vi "ex_TreeUpdateValues.vi"(4 "error in (no error)":errorcluster, 7 "Data Object in":refnum<k20>) -> (0 "error out":errorcluster, 1 "Dynamic Data":dynamicdata(waveform), 2 "Values as String array":string[][](array[string]), 3 "Header strings":string[](array[string]))   [LabVIEW 2017]
uses:
  <vilib>/Platform/storage/Storage.llb/Get Property (Storage Refnums).vi
  <vilib>/Platform/storage/Storage.llb/Get Property (Enum).vi
  <vilib>/Platform/storage/lvStorage.llb/_loadWaveform.vi
  <vilib>/Platform/storage/lvStorage.llb/xStorage/xStorageSupp/ErrorOut.vi
  <vilib>/Waveform/WDTOps.llb/WDT Waveform to XY Pairs DBL.vi
  <vilib>/Platform/storage/Storage.llb/Get Property (String).vi
  <vilib>/Platform/storage/Storage.llb/__loadStringChannel.vi
  <vilib>/Platform/storage/Storage.llb/__loadDateTimeChannel.vi
  <vilib>/Platform/storage/lvStorage.llb/xStorage/Get Properties/Get Properties.xnode
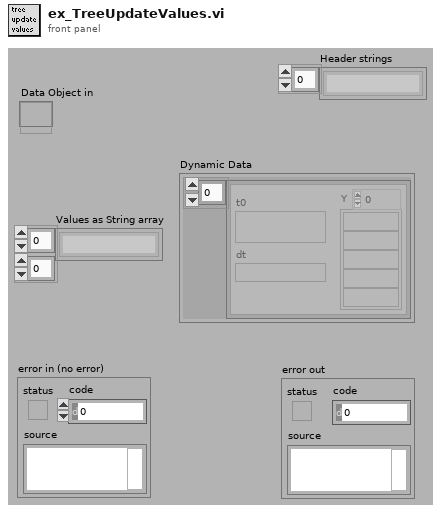
[diagram p1: front panel]
types:
  T1 = enum16{"UPDATE", "READ", "QUERY", "CREATE CHILD", "CREATE", "CONNECT", "DISCONNECT"}
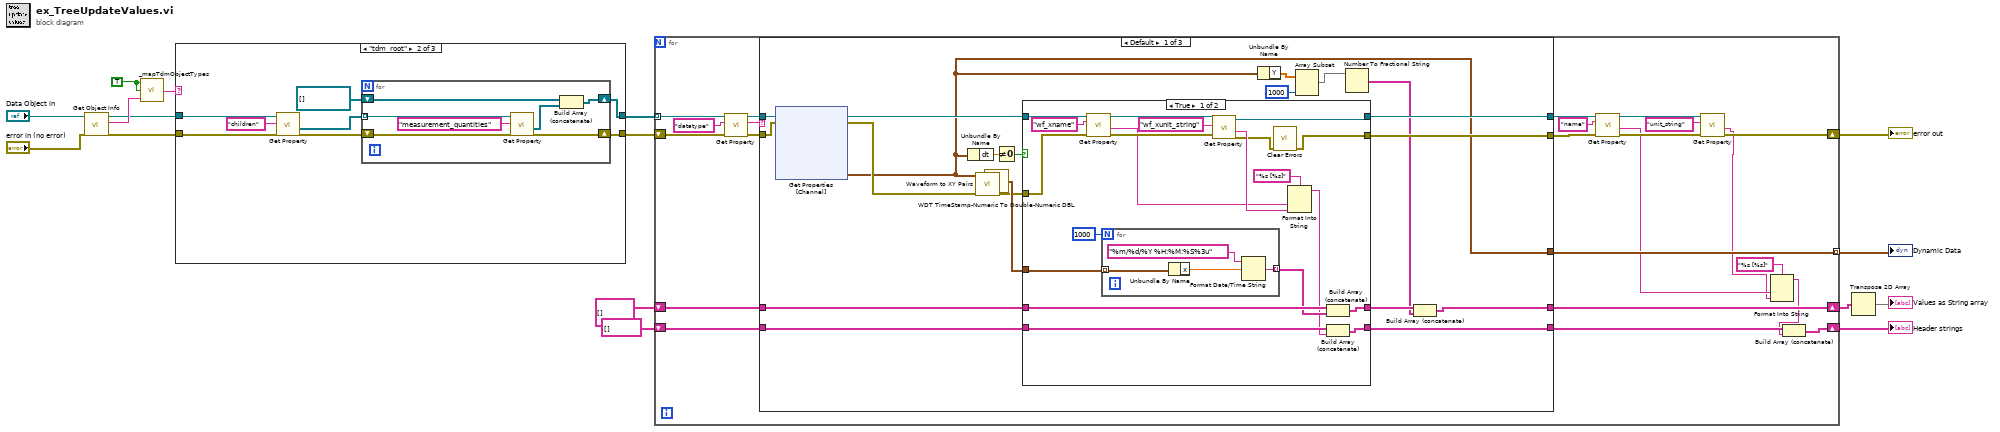
[diagram p0: block diagram]
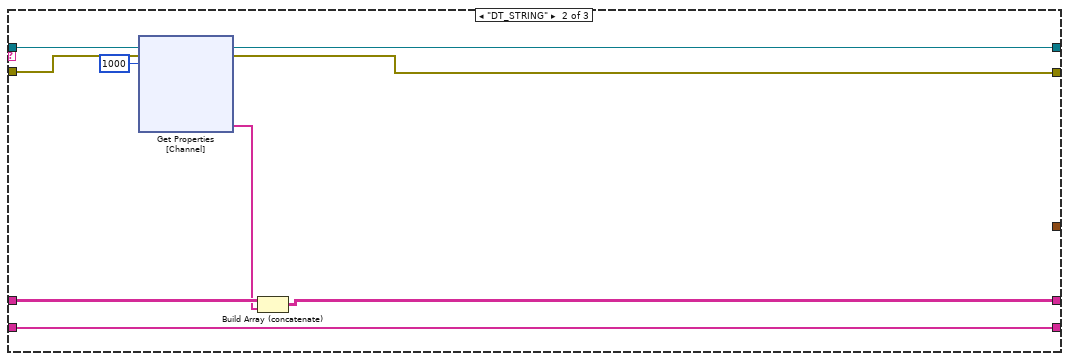
[diagram p3: hidden frame]
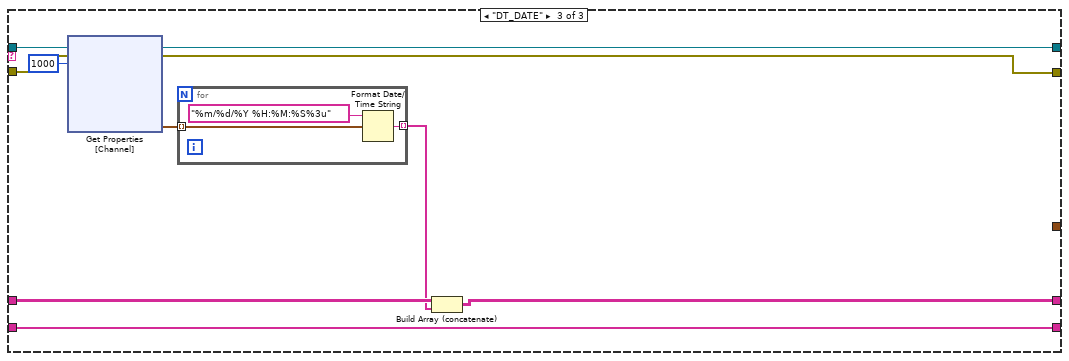
[diagram p4: hidden frame]
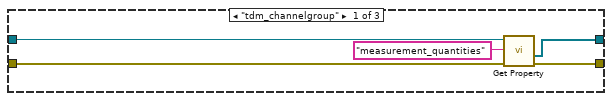
[diagram p5: hidden frame]
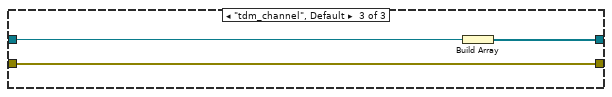
[diagram p6: hidden frame]
diagram:
  w12 = TRUE ("DNL_UnMap?(F)")
  n1 = call <vilib>:"Get Object Info.vi"("error in (no error)"="error in (no error)", "storage refnum"="Data Object in") -> ("error out"=w10:errorcluster, "object type"=w13:string, "storage refnum out"=w8:refnum<k20>)  [unwired: 7 out]
  n2 = call <vilib>:"_mapTdmObjectTypes.vi"(1:w13, "isTdmDataStructure?"=w12, "DNL_UnMap?(F)"=w12) -> (0:w11:string)
  n3 = case shown="\"tdm_root\"" w11 {
    tunnel: w10 -> [w21 w27 w39]
    tunnel: [w19 w29 w39] -> w9
    tunnel: w8 -> [w20 w26 w38]
    tunnel: [w18 w22 w37] -> w6
    frame "tdm_channelgroup" {
      n4 = call-poly <vilib>:"Get Property.vi"("error in (no error)"=w21, "Property name"="measurement_quantities", "storage refnum"=w20) -> ("error out"=w19:errorcluster, "Value"=w18:refnum<k20>[])  [unwired: 7 out]
    }
    frame "tdm_root" {
      n5 = call-poly <vilib>:"Get Property.vi"("error in (no error)"=w27, "Property name"="children", "storage refnum"=w26) -> ("error out"=w25:errorcluster, "Value"=w24:refnum<k20>[])  [unwired: 7 out]
      n6 = for {
        tunnel: w24 -> [w33] mode=indexing
        shift-right: [w30] -> w22
        shift-left: refnum<k20>[] [] ("Value") -> [w32]
        shift-right: [w36] -> w29
        shift-left: w25 -> [w34]
        n7 = call-poly <vilib>:"Get Property.vi"("error in (no error)"=w34, "Property name"="measurement_quantities", "storage refnum"=w33) -> ("error out"=w36:errorcluster, "Value"=w31:refnum<k20>[])  [unwired: 7 out]
        n8 = Build Array (concatenate)(w32, w31) -> (w30:refnum<k20>[])
      }
    }
    frame "tdm_channel", Default {
      n9 = Build Array(w38) -> (w37:refnum<k20>[])
    }
  }
  n10 = for {
    tunnel: [w62] -> w16 mode=indexing
    shift-right: [w44] -> w7
    shift-left: w9 -> [w61]
    tunnel: w6 -> [w56] mode=indexing
    shift-right: [w51] -> w4
    shift-left: string[][] [] -> [w52]
    shift-right: [w48] -> w1
    shift-left: string[] [] -> [w50]
    n11 = call-poly <vilib>:"Get Property.vi"("error in (no error)"=w61, "Property name"="datatype" ("PropertyName"), "storage refnum"=w56) -> ("error out"=w60:errorcluster, "String"=w57:string, "storage refnum out"=w59:refnum<k20>)  [unwired: 6 out]
    n12 = case shown="Default" w57 {
      tunnel: w60 -> [w76 w129 w148]
      tunnel: w59 -> [w77 w128 w147]
      tunnel: [w73 _ _] -> w62
      tunnel: [w79 w127 w146] -> w53
      tunnel: [w78 w126 w145] -> w54
      tunnel: w52 -> [w72 w125 w143]
      tunnel: [w69 w123 w141] -> w51
      tunnel: w50 -> [w65 w121 w139]
      tunnel: [w64 w121 w139] -> w49
      frame Default {
        n13 = xnode "Get Properties\n[Channel]"("storage refnum"=w77, "error in"=w76) -> ("Signal"=w73:waveform(dbl), "storage refnum out"=w75:refnum<k20>, "error out"=w74:errorcluster)  [unwired: 2 out]
        n14 = Unbundle By Name(w73) -> ("dt"=w82:dbl)
        n15 = call-poly <vilib>:"Waveform to XY Pairs.vi"("error in (no error)"=w74, "waveform in"=w73) -> ("error out"=w80:errorcluster, "XY pairs"=w63:cluster{"x":timestamp, "y":dbl}[])  [unwired: 8 out]
        n16 = call <vilib>:"WDT TimeStamp-Numeric To Double-Numeric DBL.vi"("XY pairs w/timestamp time"=w63) -> ("XY pairs w/double time"=w83:cluster{"x":dbl, "y":dbl}[])
        n17 = Not Equal To 0?(x=w82) -> (x != 0?=w81:bool)
        n18 = case shown="True" w81 {
          tunnel: w83 -> [w112 _]
          tunnel: w75 -> [w102 w120]
          tunnel: w80 -> [w101 w119]
          tunnel: [w97 w120] -> w79
          tunnel: [w93 w119] -> w78
          tunnel: w72 -> [w110 w118]
          tunnel: [w111 w118] -> w71
          tunnel: w65 -> [w107 w117]
          tunnel: [w106 w117] -> w64
          frame True {
            n19 = call-poly <vilib>:"Get Property.vi"("error in (no error)"=w101, "Property name"="wf_xname" ("PropertyName"), "storage refnum"=w102) -> ("error out"=w100:errorcluster, "Value"=w95:string, "storage refnum out"=w99:refnum<k20>)  [unwired: 6 out]
            n20 = for {
              N: 1000 -> [_]
              tunnel: w112 -> [w116] mode=indexing
              tunnel: [w113] -> w109 mode=indexing
              n21 = Unbundle By Name(w116) -> ("x"=w114:dbl)
              n22 = Format Date/Time String(time format string (%c)="%m/%d/%Y %H:%M:%S%3u", seconds (now)=w114) -> (date/time string=w113:string)  [unwired: 1 out]
            }
            n23 = call-poly <vilib>:"Get Property.vi"("error in (no error)"=w100, "Property name"="wf_xunit_string" ("PropertyName"), "storage refnum"=w99) -> ("error out"=w94:errorcluster, "Value"=w96:string, "storage refnum out"=w97:refnum<k20>)  [unwired: 6 out]
            n24 = call <vilib>:"Clear Errors.vi"("error in (no error)"=w94) -> ("error out"=w93:errorcluster)  [unwired: 1 in, 5 out]
            n25 = Format Into String(format string="%s [%s]", w95, w96) -> (resulting string=w104:string)  [unwired: 2 in, 1 out]
            n26 = Build Array (concatenate)(w110, w109) -> (w111:string[][])
            n27 = Build Array (concatenate)(w107, w104) -> (w106:string[])
          }
          frame False {
          }
        }
        n28 = Unbundle By Name(w73) -> ("Y"=w68:dbl[])
        n29 = Array Subset(array=w68, length=1000) -> (w67:dbl[])  [unwired: 1 in]
        n30 = Number To Fractional String(number=w67) -> (F-format string=w70:string[])  [unwired: 3 out]
        n31 = Build Array (concatenate)(w71, w70) -> (w69:string[][])
      }
      frame "DT_STRING" {
        n32 = xnode "Get Properties\n[Channel]"("storage refnum"=w128, "error in"=w129, "count"=1000) -> ("Signal"=w124:string[], "storage refnum out"=w127:refnum<k20>, "error out"=w126:errorcluster)  [unwired: 1 out]
        n33 = Build Array (concatenate)(w125, w124) -> (w123:string[][])
      }
      frame "DT_DATE" {
        n34 = xnode "Get Properties\n[Channel]"("storage refnum"=w147, "error in"=w148, "count"=1000) -> ("Signal"=w144:timestamp[], "storage refnum out"=w146:refnum<k20>, "error out"=w145:errorcluster)  [unwired: 1 out]
        n35 = for {
          tunnel: w144 -> [w160] mode=indexing
          tunnel: [w158] -> w142 mode=indexing
          n36 = Format Date/Time String(time format string (%c)="%m/%d/%Y %H:%M:%S%3u", seconds (now)=w160) -> (date/time string=w158:string)  [unwired: 1 out]
        }
        n37 = Build Array (concatenate)(w143, w142) -> (w141:string[][])
      }
    }
    n38 = call-poly <vilib>:"Get Property.vi"("error in (no error)"=w54, "Property name"="name" ("PropertyName"), "storage refnum"=w53) -> ("error out"=w47:errorcluster, "Value"=w42:string, "storage refnum out"=w46:refnum<k20>)  [unwired: 6 out]
    n39 = call-poly <vilib>:"Get Property.vi"("error in (no error)"=w47, "Property name"="unit_string" ("PropertyName"), "storage refnum"=w46) -> ("error out"=w44:errorcluster, "Value"=w41:string)  [unwired: 7 out]
    n40 = Format Into String(format string="%s [%s]", w42, w41) -> (resulting string=w40:string)  [unwired: 2 in, 1 out]
    n41 = Build Array (concatenate)(w49, w40) -> (w48:string[])
  }
  "Dynamic Data" <- w16
  "error out" <- w7
  "Header strings" <- w1
  n42 = Transpose 2D Array(2D array=w4) -> (transposed array=→"Values as String array":string[][])
